vi "流程批量写入.vi"(10 "简易流程路径":path, 11 "添加的路径":path caption="测试流程路径") -> ()   [LabVIEW 2016, in "斯坦道总磷.lvlib"]
uses:
  <vilib>/Utility/miscctls.llb/LVPointTypeDef.ctl
panel:
  in  "校验":bool
  in  "选项卡控件":enum32{"测试流程", "简易流程"}(tab)
  in  "一键写入":bool
  in  "量程下拉列表":enum16{"低量程", "高量程"}(ring)
  in  "测量模式":T1(ring)
  in  "简易流程":u16(ring)
  in  "一键写入 2":bool=TRUE
  in  "关闭":bool
  out "字符串":string
  in  "写入":bool
  in  "参数下拉列表":u16(ring)
  # "请选择要写入的流程"
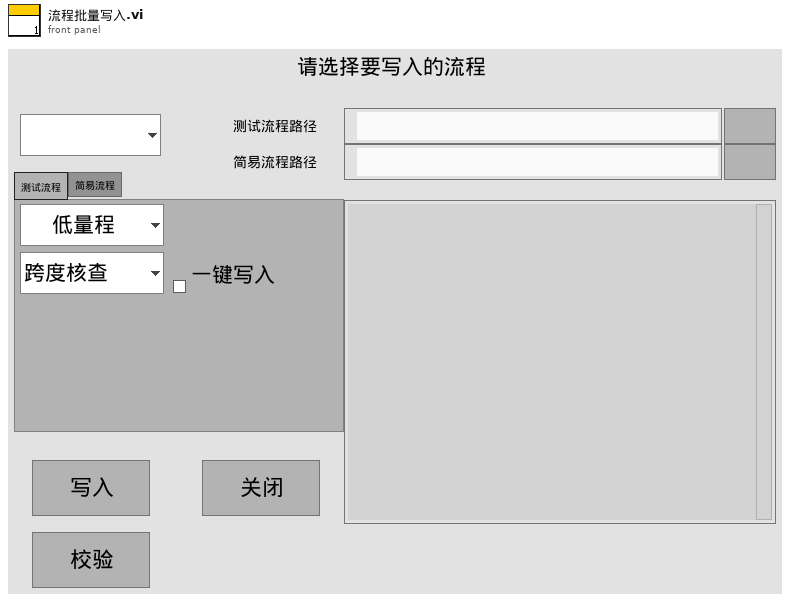
[diagram p1: front panel]
types:
  T1 = enum16{"跨度核查", "水样测量", "零点核查", "标样核查", "加标回收", "快捷测试", "空白校准", "标样校准"}
  T2 = typedef "LVPointTypeDef.ctl" = cluster{"Horizontal":i16, "Vertical":i16}
  T3 = typedef "LVStringsAndValuesArrayTypeDef_U16.ctl" = cluster{"String":string, "Value":u16}[]
  T4 = typedef "操作日志字段定义.ctl" = cluster{"时间":timestamp, "参数":string, "日志信息":string, "流程参数":string}
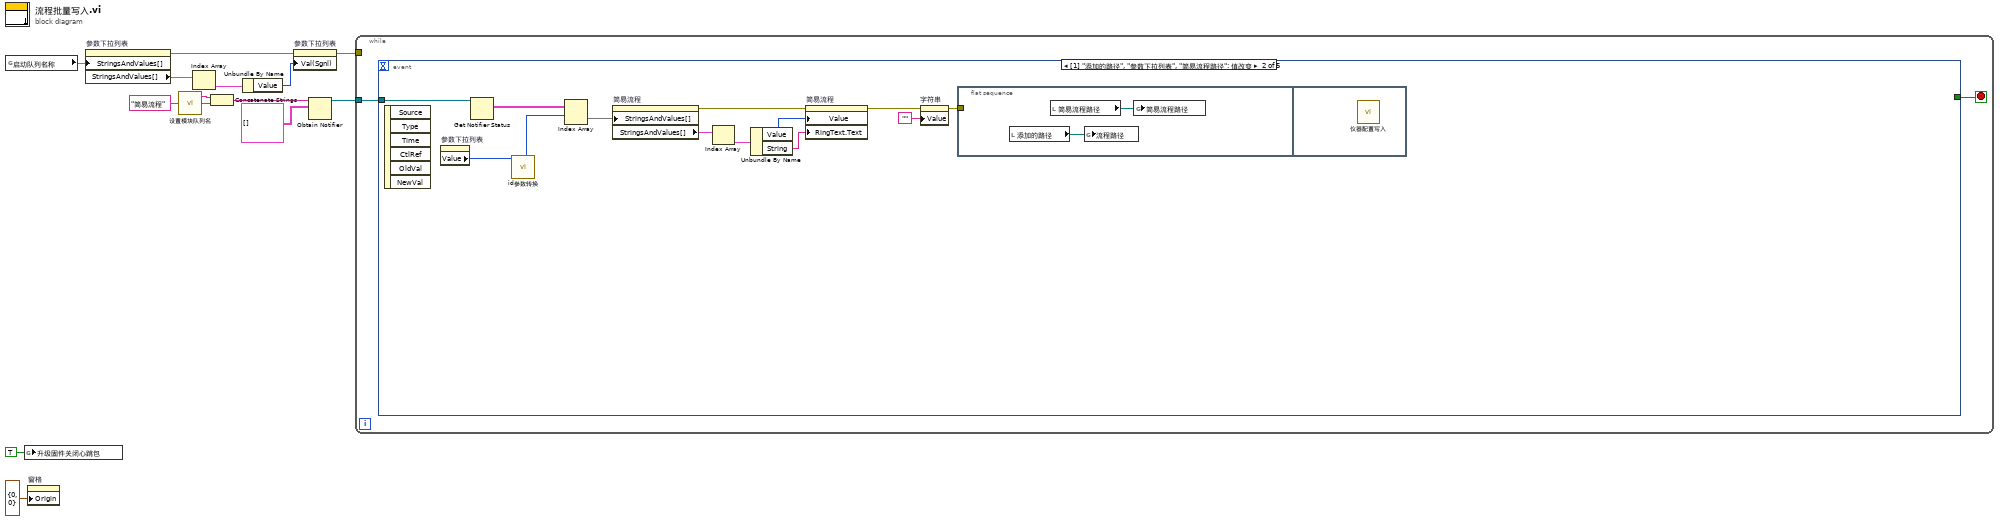
[diagram p0: block diagram]
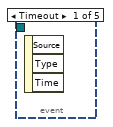
[diagram p2: hidden frame]
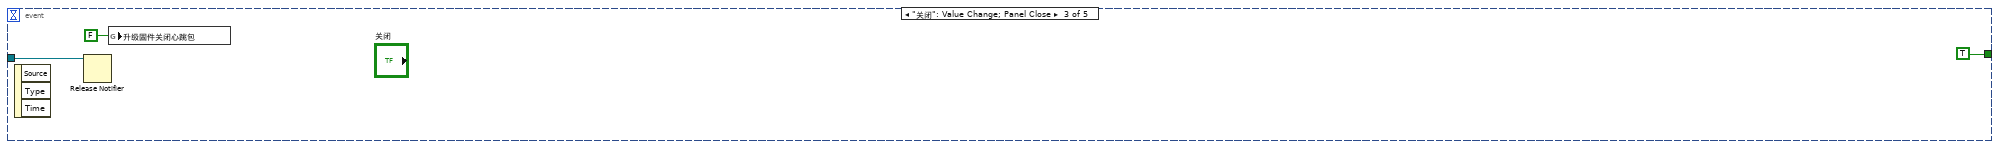
[diagram p3: hidden frame]
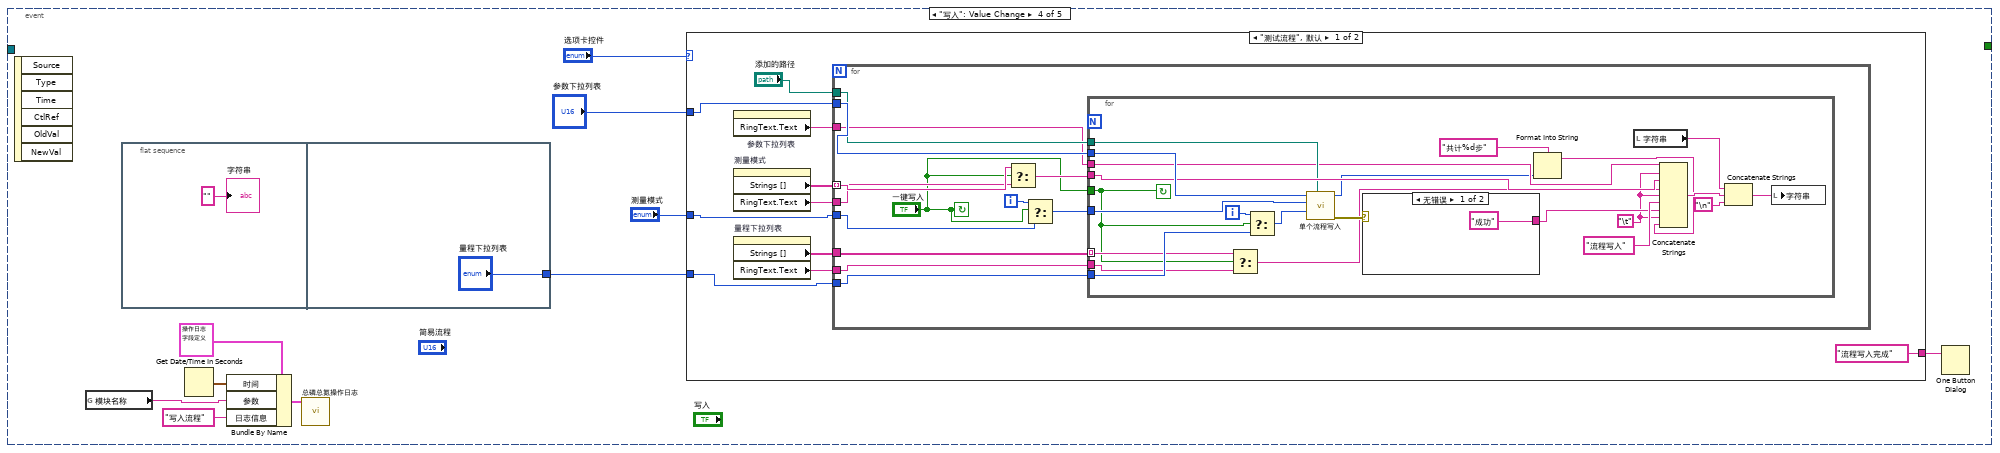
[diagram p4: hidden frame]
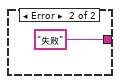
[diagram p5: hidden frame]
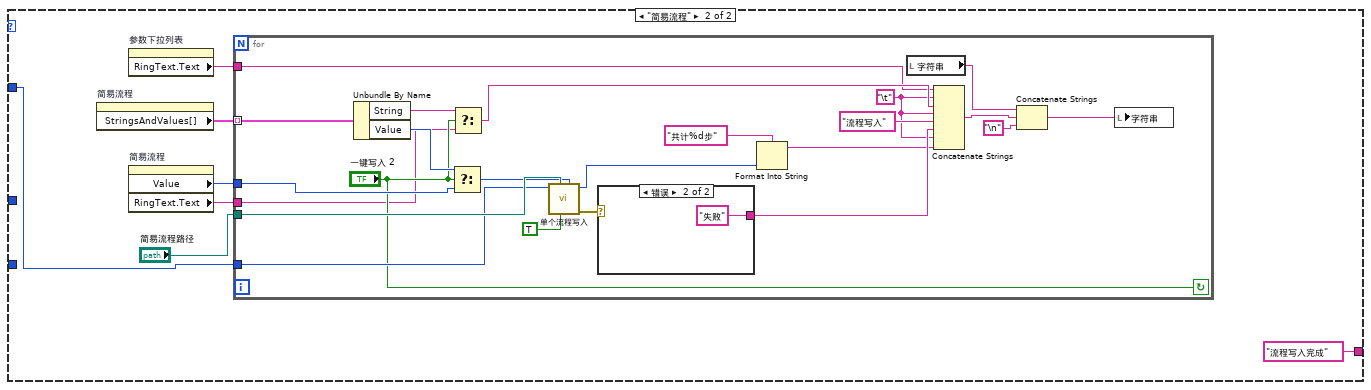
[diagram p6: hidden frame]
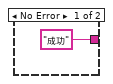
[diagram p7: hidden frame]
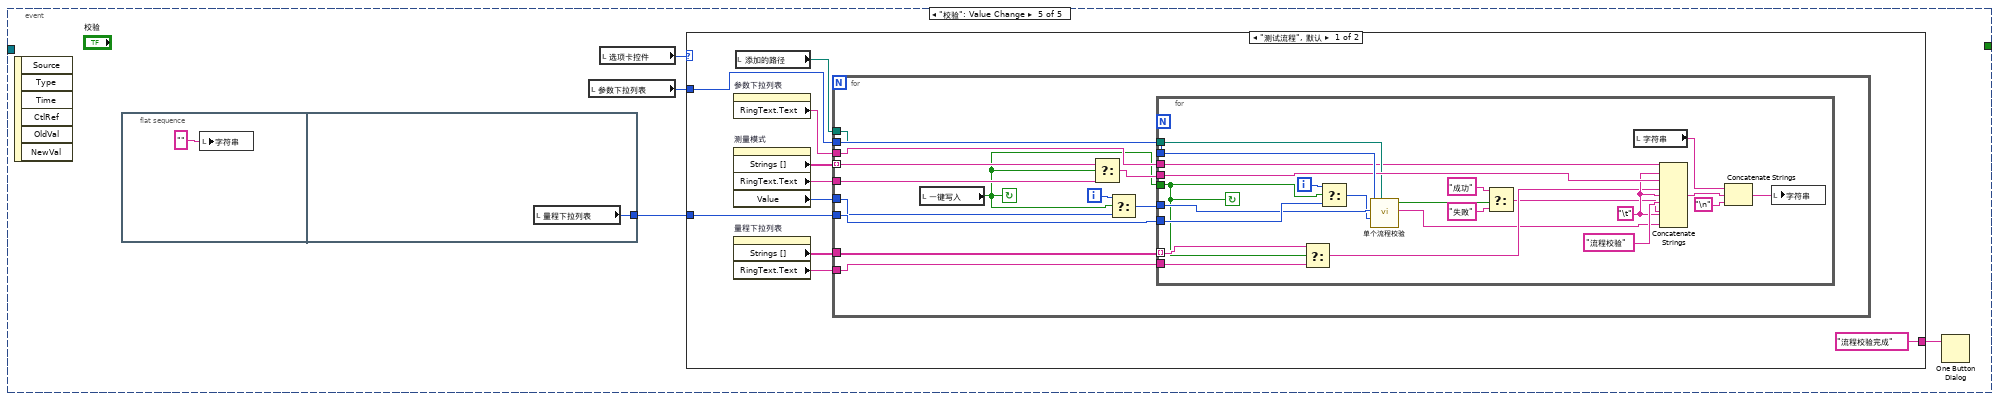
[diagram p8: hidden frame]
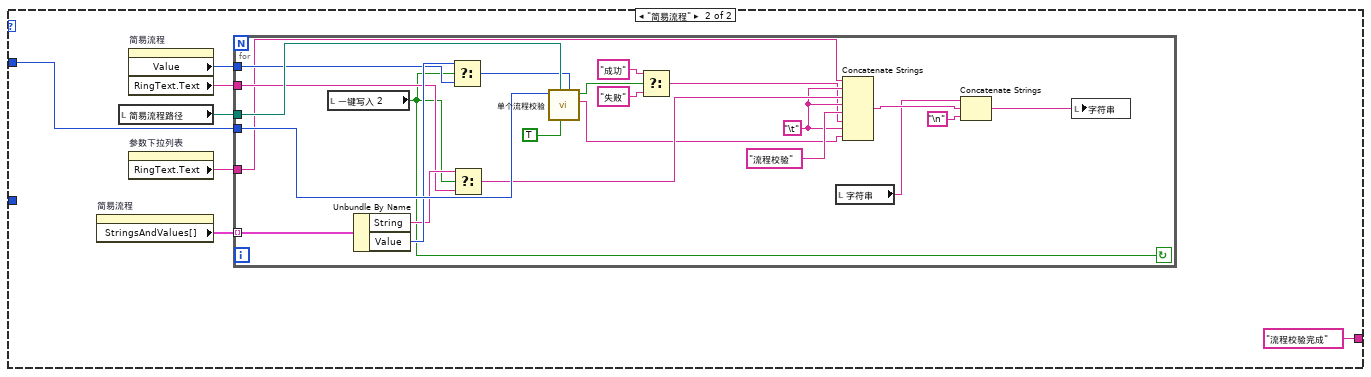
[diagram p9: hidden frame]
diagram:
  n1 = global read "model config var.vi" "启动队列名称"() -> (w12:cluster{"String":string, "Value":u16}[])
  n2 = global write "VAR总磷总氮全局变量.vi" "升级固件关闭心跳包"(TRUE ("升级固件关闭心跳包")) -> ()
  n3 = property on="窗格" class="Pane"("Origin"=T2 {"Horizontal"=0, "Vertical"=0} ("原点")) -> ()  [unwired: 2 in, 2 out]
  n4 = property on="参数下拉列表" class="Ring (严格)"("StringsAndValues[]"=w12) -> (error out=w11:errorcluster, "StringsAndValues[]"=w10:T3)  [unwired: 2 in, 1 out]
  n5 = call "设置模块队列名.vi"() -> ("Msg"=w4:string)  [unwired: 5 in]
  n6 = Index Array(array=w10) -> (element=w9:cluster{"String":string, "Value":u16})  [unwired: 1 in]
  n7 = Concatenate Strings(w4, "简易流程" ("Msg")) -> (w2:string)
  n8 = Unbundle By Name(w9) -> ("Value"=w8:u16)
  n9 = property on="参数下拉列表" class="Ring (严格)"(error in=w11, "Val(Sgnl)"=w8) -> (error out=w7:errorcluster)  [unwired: 1 in, 1 out]
  n10 = Obtain Notifier(name (unnamed)=w2, notification data type=cluster{string, i32}[][] [] ("数组")) -> (notifier out=w1:refnum<notifier>)  [unwired: 2 in, 2 out]
  n11 = while {
    tunnel: w7 -> [_]
    tunnel: w1 -> [w14]
    stop <- w15 stop-if-true
    n12 = event shown="[1] \"添加的路径\", \"参数下拉列表\", \"简易流程路径\": 值改变" {
      selector: _ -> [_ _ _ _ _]
      dyn-events: _ -> [_ _ _ _ _]
      timeout: _ -> [_ _ _ _ _]
      tunnel: [_ _ TRUE _ _] -> w15
      tunnel: w14 -> [_ w20 w31 _ _]
      event Timeout {
        n13 = event-data() -> ()  [unwired: 1 in, 3 out]
      }
      event "添加的路径", "参数下拉列表", "简易流程路径": Value Change {
        n14 = event-data() -> ()  [unwired: 1 in, 6 out]
        n15 = property on="参数下拉列表" class="Ring (严格)"() -> ("Value"=w17:u16)  [unwired: 2 in, 2 out]
        n16 = Get Notifier Status(notifier=w20) -> (current notification=w19:cluster{string, i32}[][])  [unwired: 1 in, 4 out]
        n17 = call "id参数转换.vi"("id"=w17) -> ("数组资源索引"=w16:i32)  [unwired: 9 in, 1 out]
        n18 = Index Array(array=w19, index (row)=w16) -> (element=w18:cluster{string, i32}[])  [unwired: 1 in]
        n19 = property on="简易流程" class="Ring (严格)"("StringsAndValues[]"=w18) -> (error out=w27:errorcluster, "StringsAndValues[]"=w25:T3)  [unwired: 2 in, 1 out]
        n20 = Index Array(array=w25) -> (element=w24:cluster{"String":string, "Value":u16})  [unwired: 1 in]
        n21 = Unbundle By Name(w24) -> ("Value"=w23:u16, "String"=w21:string)
        n22 = property on="简易流程" class="Ring (严格)"(error in=w27, "Value"=w23, "RingText.Text"=w21) -> (error out=w26:errorcluster)  [unwired: 1 in, 1 out]
        n23 = property on="字符串" class="Str"(error in=w26, "Value"="") -> (error out=w22:errorcluster)  [unwired: 1 in, 1 out]
        n24 = flat-sequence {
          tunnel: w22 -> [_]
          frame #0 {
            n25 = local read "添加的路径"() -> (w29:path)
            n26 = local read "简易流程路径"() -> (w30:path)
            n27 = global write "总磷总氮断电保存全局变量.vi" "流程路径"(w29) -> ()
            n28 = global write "总磷总氮断电保存全局变量.vi" "简易流程路径"(w30) -> ()
          }
          frame #1 {
            n29 = call "仪器配置写入.vi"() -> ()  [unwired: 11 in, 1 out]
          }
        }
      }
      event "关闭": Value Change; Panel Close {
        n30 = event-data() -> ()  [unwired: 1 in, 3 out]
        n31 = Release Notifier(notifier=w31) -> ()  [unwired: 2 in, 3 out]
        n32 = global write "VAR总磷总氮全局变量.vi" "升级固件关闭心跳包"(FALSE ("升级固件关闭心跳包")) -> ()
      }
      event "写入": Value Change {
        n33 = event-data() -> ()  [unwired: 1 in, 6 out]
        n34 = global read "VAR总磷总氮全局变量.vi" "模块名称"() -> (w34:string)
        n35 = flat-sequence {
          tunnel: ["量程下拉列表"] -> w42
          frame #0 {
            "字符串" <- ""
          }
          frame #1 {
          }
        }
        n36 = Get Date/Time In Seconds() -> (seconds since 1Jan1904=w36:timestamp)
        n37 = Bundle By Name(cluster=T4 {"时间"=timestamp(0 s since 1904-01-01), "参数"="", "日志信息"="", "流程参数"=""} ("data in"), "时间"=w36, "参数"=w34, "日志信息"="写入流程") -> (w37:T4)
        n38 = call "总磷总氮操作日志.vi"("data in"=w37) -> ()  [unwired: 10 in, 1 out]
        n39 = case shown="\"测试流程\", 默认" "选项卡控件" {
          tunnel: "参数下拉列表" -> [w51 w98]
          tunnel: w42 -> [w52 _]
          tunnel: ["流程写入完成" ("消息") "流程写入完成" ("消息")] -> w40
          tunnel: "测量模式" -> [w49 _]
          frame "测试流程", Default {
            n40 = property on="参数下拉列表" class="Ring (严格)"() -> ("RingText.Text"=w46:string)  [unwired: 2 in, 2 out]
            n41 = property on="测量模式" class="Enum (严格)"() -> ("Strings []"=w50:string[], "RingText.Text"=w47:string)  [unwired: 2 in, 2 out]
            n42 = property on="量程下拉列表" class="Enum (严格)"() -> ("Strings []"=w44:string[], "RingText.Text"=w48:string)  [unwired: 2 in, 2 out]
            n43 = for {
              tunnel: w52 -> [w66]
              tunnel: w51 -> [w64]
              tunnel: w50 -> [w60] mode=indexing
              tunnel: w49 -> [w63]
              tunnel: w48 -> [w61]
              tunnel: w47 -> [w59]
              tunnel: "添加的路径" -> [w57]
              tunnel: w46 -> [w56]
              tunnel: w44 -> [w54]
              i -> [w65]
              stop <- "一键写入" continue-if-true
              n44 = Select(t=w60, s="一键写入", f=w59) -> (s? t:f=w58:string)
              n45 = Select(t=w65, s="一键写入", f=w63) -> (s? t:f=w62:i32)
              n46 = for {
                tunnel: w66 -> [w82]
                tunnel: w64 -> [w81]
                tunnel: w62 -> [w80]
                tunnel: w61 -> [w69]
                tunnel: w58 -> [w79]
                tunnel: w57 -> [w78]
                tunnel: w56 -> [w77]
                tunnel: "一键写入" -> [w67]
                tunnel: w54 -> [w70] mode=indexing
                i -> [w71]
                stop <- w67 continue-if-true
                w73 = "\t"
                n47 = Select(t=w70, s=w67, f=w69) -> (s? t:f=w68:string)
                n48 = Select(t=w71, s=w67, f=w82) -> (s? t:f=w72:i32)
                n49 = call "单个流程写入.vi"("添加的路径"=w78, "量程"=w72, "测量模式"=w80, "测量参数"=w81) -> ("error out"=w89:errorcluster, "大小"=w76:i32)  [unwired: 6 in]
                n50 = case shown="无错误" w89 {
                  tunnel: ["成功" "失败"] -> w86
                  frame No Error {
                  }
                  frame Error {
                  }
                }
                n51 = Format Into String(format string="共计%d步" ("格式字符串"), w76) -> (resulting string=w74:string)  [unwired: 2 in, 1 out]
                n52 = local read "字符串"() -> (w88:string)
                n53 = Concatenate Strings(w77, w73, w79, w68, w73, "流程写入", w86, w73, w74) -> (w85:string)
                n54 = Concatenate Strings(w88, w85, "\n") -> (w83:string)
                n55 = local write "字符串"(w83) -> ()
              }
            }
          }
          frame "简易流程" {
            n56 = property on="简易流程" class="Ring (严格)"() -> ("StringsAndValues[]"=w97:T3)  [unwired: 2 in, 2 out]
            n57 = property on="参数下拉列表" class="Ring (严格)"() -> ("RingText.Text"=w92:string)  [unwired: 2 in, 2 out]
            n58 = property on="简易流程" class="Ring (严格)"() -> ("Value"=w95:u16, "RingText.Text"=w94:string)  [unwired: 2 in, 2 out]
            n59 = for {
              tunnel: w97 -> [w111] mode=indexing
              tunnel: "简易流程路径" -> [w114]
              tunnel: w98 -> [w113]
              tunnel: w95 -> [w108]
              tunnel: w94 -> [w105]
              tunnel: w92 -> [w99]
              stop <- "一键写入 2" continue-if-true
              w100 = "\t"
              n60 = Unbundle By Name(w111) -> ("String"=w106:string, "Value"=w110:u16)
              n61 = Select(t=w110, s="一键写入 2", f=w108) -> (s? t:f=w109:u16)
              n62 = Select(t=w106, s="一键写入 2", f=w105) -> (s? t:f=w104:string)
              n63 = call "单个流程写入.vi"("简易流程Id"=w109, "是否是简易流程"=TRUE, "添加的路径"=w114, "测量参数"=w113) -> ("error out"=w121:errorcluster, "大小"=w103:i32)  [unwired: 6 in]
              n64 = case shown="错误" w121 {
                tunnel: ["成功" "失败"] -> w118
                frame No Error {
                }
                frame Error {
                }
              }
              n65 = Format Into String(format string="共计%d步" ("格式字符串"), w103) -> (resulting string=w101:string)  [unwired: 2 in, 1 out]
              n66 = local read "字符串"() -> (w120:string)
              n67 = Concatenate Strings(w99, w100, w104, w100, "流程写入", w118, w100, w101) -> (w117:string)
              n68 = Concatenate Strings(w120, w117, "\n") -> (w115:string)
              n69 = local write "字符串"(w115) -> ()
            }
          }
        }
        n70 = One Button Dialog(message=w40) -> ()  [unwired: 1 in, 1 out]
      }
      event "校验": Value Change {
        n71 = event-data() -> ()  [unwired: 1 in, 6 out]
        n72 = flat-sequence {
          tunnel: [w207] -> w129
          frame #0 {
            n73 = local write "字符串"("") -> ()
          }
          frame #1 {
            n74 = local read "量程下拉列表"() -> (w207:enum16{"低量程", "高量程"})
          }
        }
        n75 = local read "参数下拉列表"() -> (w126:u16)
        n76 = local read "选项卡控件"() -> (w127:enum32{"测试流程", "简易流程"})
        n77 = case shown="\"测试流程\", 默认" w127 {
          tunnel: w126 -> [w137 w182]
          tunnel: w129 -> [w138 _]
          tunnel: ["流程校验完成" ("消息") "流程校验完成" ("消息")] -> w128
          frame "测试流程", Default {
            n78 = property on="参数下拉列表" class="Ring (严格)"() -> ("RingText.Text"=w133:string)  [unwired: 2 in, 2 out]
            n79 = property on="测量模式" class="Enum (严格)"() -> ("Strings []"=w136:string[], "RingText.Text"=w134:string, "Value"=w130:T1)  [unwired: 2 in, 2 out]
            n80 = property on="量程下拉列表" class="Enum (严格)"() -> ("Strings []"=w132:string[], "RingText.Text"=w135:string)  [unwired: 2 in, 2 out]
            n81 = local read "添加的路径"() -> (w131:path)
            n82 = for {
              tunnel: w138 -> [w152]
              tunnel: w137 -> [w150]
              tunnel: w136 -> [w146] mode=indexing
              tunnel: w130 -> [w149]
              tunnel: w135 -> [w147]
              tunnel: w134 -> [w145]
              tunnel: w131 -> [w143]
              tunnel: w133 -> [w142]
              tunnel: w132 -> [w141]
              i -> [w151]
              stop <- w140 continue-if-true
              n83 = local read "一键写入"() -> (w140:bool)
              n84 = Select(t=w146, s=w140, f=w145) -> (s? t:f=w144:string)
              n85 = Select(t=w151, s=w140, f=w149) -> (s? t:f=w148:i32)
              n86 = for {
                tunnel: w152 -> [w172]
                tunnel: w150 -> [w171]
                tunnel: w148 -> [w170]
                tunnel: w147 -> [w162]
                tunnel: w144 -> [w169]
                tunnel: w143 -> [w168]
                tunnel: w142 -> [w167]
                tunnel: w140 -> [w153]
                tunnel: w141 -> [w163] mode=indexing
                i -> [w164]
                stop <- w153 continue-if-true
                w166 = "\t"
                n87 = Select(t=w163, s=w153, f=w162) -> (s? t:f=w161:string)
                n88 = Select(t=w164, s=w153, f=w172) -> (s? t:f=w165:i32)
                n89 = call "单个流程校验.vi"("添加的路径"=w168, "量程"=w165, "测量模式"=w170, "测量参数"=w171) -> ("结果字符串"=w154:string, "check？"=w155:bool)  [unwired: 5 in, 1 out]
                n90 = Select(t="成功", s=w155, f="失败") -> (s? t:f=w156:string)
                n91 = local read "字符串"() -> (w160:string)
                n92 = Concatenate Strings(w167, w166, w169, w161, w166, "流程校验", w156, w166, w154) -> (w174:string)
                n93 = Concatenate Strings(w160, w174, "\n") -> (w159:string)
                n94 = local write "字符串"(w159) -> ()
              }
            }
          }
          frame "简易流程" {
            n95 = property on="简易流程" class="Ring (严格)"() -> ("StringsAndValues[]"=w181:T3)  [unwired: 2 in, 2 out]
            n96 = local read "简易流程路径"() -> (w176:path)
            n97 = property on="简易流程" class="Ring (严格)"() -> ("Value"=w179:u16, "RingText.Text"=w178:string)  [unwired: 2 in, 2 out]
            n98 = property on="参数下拉列表" class="Ring (严格)"() -> ("RingText.Text"=w177:string)  [unwired: 2 in, 2 out]
            n99 = for {
              tunnel: w181 -> [w199] mode=indexing
              tunnel: w176 -> [w202]
              tunnel: w182 -> [w201]
              tunnel: w179 -> [w196]
              tunnel: w178 -> [w194]
              tunnel: w177 -> [w191]
              stop <- w190 continue-if-true
              w192 = "\t"
              n100 = local read "一键写入 2"() -> (w190:bool)
              n101 = Unbundle By Name(w199) -> ("String"=w195:string, "Value"=w198:u16)
              n102 = Select(t=w198, s=w190, f=w196) -> (s? t:f=w197:u16)
              n103 = Select(t=w195, s=w190, f=w194) -> (s? t:f=w193:string)
              n104 = call "单个流程校验.vi"("简易流程Id"=w197, "是否是简易流程"=TRUE, "添加的路径"=w202, "测量参数"=w201) -> ("结果字符串"=w183:string, "check？"=w184:bool)  [unwired: 5 in, 1 out]
              n105 = Select(t="成功", s=w184, f="失败") -> (s? t:f=w185:string)
              n106 = local read "字符串"() -> (w189:string)
              n107 = Concatenate Strings(w191, w192, w193, w192, "流程校验", w185, w192, w183) -> (w204:string)
              n108 = Concatenate Strings(w189, w204, "\n") -> (w188:string)
              n109 = local write "字符串"(w188) -> ()
            }
          }
        }
        n110 = One Button Dialog(message=w128) -> ()  [unwired: 1 in, 1 out]
      }
    }
  }
